vi "AuMT8852B CW Measurement Configuration.vi"(5 "Frequency (2441)":dbl=2441.0, 7 "Set/Get (Set)":enum16{"Set", "Get"}(ring), 8 "error in (no error)":errorcluster, 9 "Frequency units (MHz)":enum16{"Channel", "MHz"}(ring)=enum."MHz", 10 "Gate width (1 ms)":dbl=1.0 format="%.2f", 11 "VISA session":refnum<visa-resource-name>) -> (0 "error out":errorcluster, 1 "Frequency units out":enum16{"Channel", "MHz"}(ring)=enum."MHz", 2 "error code":i32, 3 "VISA session out":refnum<visa-resource-name>, 4 "Frequency out":dbl=2441.0, 6 "Gate width out":dbl=1.0 format="%.2f")   [LabVIEW 2017]
doc: "Anritsu MT8852B Bluetooth Tester\n\nSets the frequency and measurement period for the CW measurement.\n\nINPUTS\nSet/Get - whether the configuration is being sent to or retrieved from the instrument.\nFrequency - frequency at which the CW measurement will be made.\nFrequency units - whether frequency will be read/written as a channel or as a frequency in MHz.\nGate width - measurement period in ms.\n\nOUTPUTS\nFrequency out - current CW measurement frequency.\nFrequency units out - whether frequency is returned as a channel or as a frequency in MHz.\nGate width - current CW measurement period in ms."
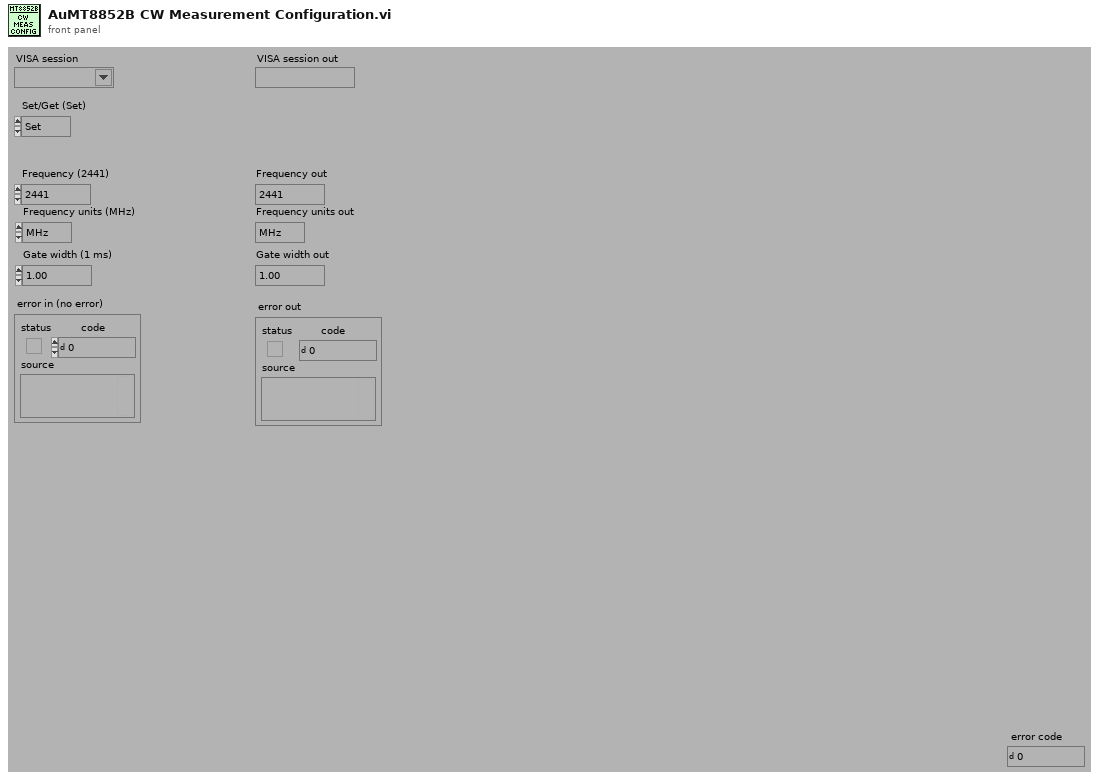
[diagram p1: front panel]
types:
  T1 = enum16{"Simulate", "Range check", "Cache", "Query instrument status"}
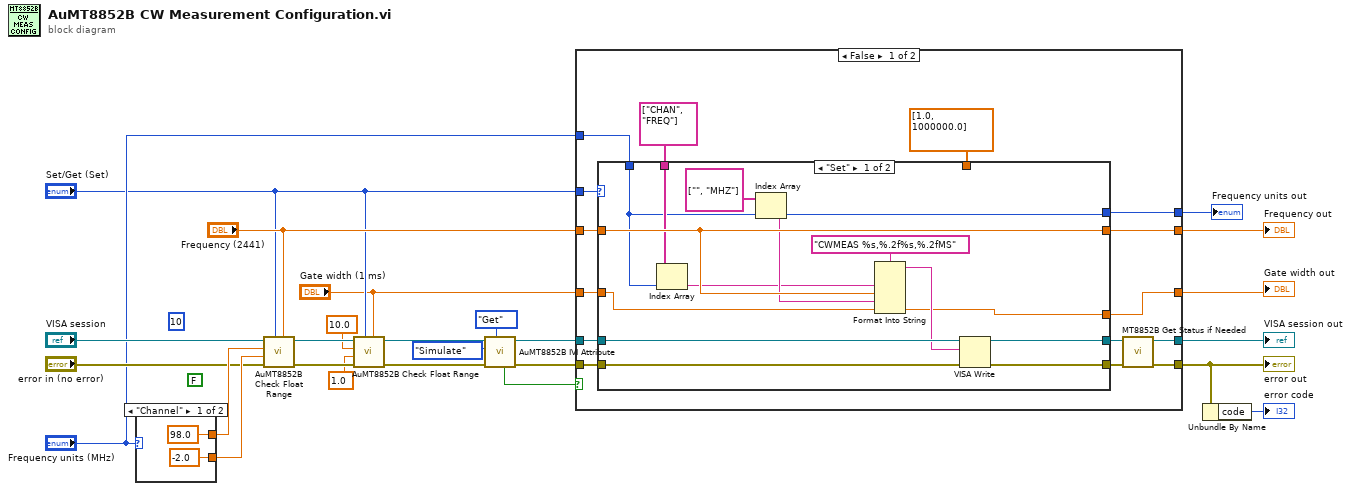
[diagram p0: block diagram]
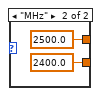
[diagram p2: hidden frame]
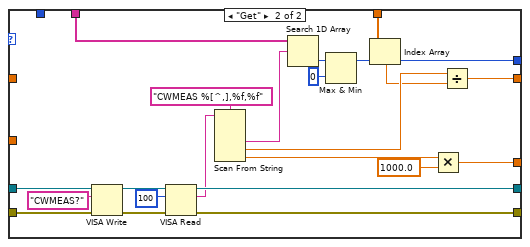
[diagram p3: hidden frame]
diagram:
  (unwired) FALSE ("Check IVI flag first? (T)")
  (unwired) 10 ("Upper limit (1)")
  n1 = case shown="\"Channel\"" "Frequency units (MHz)" {
    tunnel: [98.0 ("Upper limit (1)") 2500.0 ("Upper limit (1)")] -> w15
    tunnel: [-2.0 ("Lower limit (-1)") 2400.0 ("Lower limit (-1)")] -> w14
    frame "Channel" {
    }
    frame "MHz" {
    }
  }
  n2 = call <instrlib>:"AuMT8852B Check Float Range.vi"("Value (0)"="Frequency (2441)", "Set/Get (Set)"="Set/Get (Set)", "error in (no error)"="error in (no error)", "Lower limit (-1)"=w14, "Upper limit (1)"=w15, "VISA session"="VISA session") -> ("error out"=w9:errorcluster, "VISA session out"=w8:refnum<visa-resource-name>)  [unwired: 4 in]
  n3 = call <instrlib>:"AuMT8852B Check Float Range.vi"("Value (0)"="Gate width (1 ms)", "Set/Get (Set)"="Set/Get (Set)", "error in (no error)"=w9, "Lower limit (-1)"=1.0, "Upper limit (1)"=10.0, "VISA session"=w8) -> ("error out"=w6:errorcluster, "VISA session out"=w7:refnum<visa-resource-name>)  [unwired: 4 in]
  n4 = call <instrlib>:"AuMT8852B IVI Attribute.vi"("Set/Get (Set)"=enum16{"Set", "Get"}."Get", "error in (no error)"=w6, "Flag (Simulate)"=T1."Simulate", "VISA session"=w7) -> ("error out"=w23:errorcluster, "VISA session out"=w24:refnum<visa-resource-name>, "Value out"=w20:bool)  [unwired: 5 in]
  n5 = case shown="False" w20 {
    tunnel: "Set/Get (Set)" -> [w44 _]
    tunnel: [w38 w83] -> w18
    tunnel: [w39 w84] -> w25
    tunnel: w24 -> [w43 w84]
    tunnel: w23 -> [w42 w83]
    tunnel: "Frequency (2441)" -> [w37 w82]
    tunnel: [w36 w82] -> w17
    tunnel: "Frequency units (MHz)" -> [w31 w80]
    tunnel: "Gate width (1 ms)" -> [w35 w81]
    tunnel: [w34 w81] -> w10
    tunnel: [w30 w80] -> w1
    frame False {
      n6 = case shown="\"Set\"" w44 {
        tunnel: [w54 w73] -> w40
        tunnel: [w55 w74] -> w41
        tunnel: w43 -> [w57 w79]
        tunnel: w42 -> [w56 w78]
        tunnel: w37 -> [w51 _]
        tunnel: [w51 w72] -> w36
        tunnel: string[] ["CHAN", "FREQ"] ("Array Constant") -> [w47 w64]
        tunnel: w35 -> [w50 _]
        tunnel: [w50 w67] -> w34
        tunnel: w31 -> [w46 _]
        tunnel: dbl[] [1.0, 1000000.0] ("Input Array") -> [_ w59]
        tunnel: [w46 w62] -> w30
        frame "Set" {
          n7 = Index Array(array=w47, index=w46) -> (element=w45:string)
          n8 = Index Array(array=string[] ["", "MHZ"] ("Array Constant"), index=w46) -> (element=w48:string)
          n9 = Format Into String(format string="CWMEAS %s,%.2f%s,%.2fMS" ("Format String"), w45, w51, w48, w50) -> (resulting string=w52:string)  [unwired: 2 in, 1 out]
          n10 = VISA Write(VISA resource name=w57, write buffer=w52, error in (no error)=w56) -> (VISA resource name out=w55:refnum<visa-resource-name>, error out=w54:errorcluster)  [unwired: 1 out]
        }
        frame "Get" {
          n11 = VISA Write(VISA resource name=w79, write buffer="CWMEAS?" ("Format String"), error in (no error)=w78) -> (VISA resource name out=w77:refnum<visa-resource-name>, error out=w75:errorcluster)  [unwired: 1 out]
          n12 = VISA Read(VISA resource name=w77, byte count=u32 100 ("byte count (0)"), error in (no error)=w75) -> (VISA resource name out=w74:refnum<visa-resource-name>, read buffer=w71:string, error out=w73:errorcluster)  [unwired: 1 out]
          n13 = Scan From String(format string="CWMEAS %[^,],%f,%f" ("Format String"), input string=w71) -> (output 1=w63:string, output 2=w69:dbl, output 3=w68:dbl)  [unwired: 5 in, 3 out]
          n14 = Search 1D Array(1D array=w64, element=w63) -> (index of element=w60:i32)  [unwired: 1 in]
          n15 = Max & Min(x=w60, y=0 ("x")) -> (max(x,y)=w62:i32)  [unwired: 1 out]
          n16 = Index Array(array=w59, index=w62) -> (element=w58:dbl)
          n17 = Multiply(x=w68, y=1000.0) -> (x*y=w67:dbl)
          n18 = Divide(x=w69, y=w58) -> (x/y=w72:dbl)
        }
      }
      n19 = call <instrlib>:"MT8852B Get Status if Needed.vi"("error in (no error)"=w40, "VISA session"=w41) -> ("error out"=w38:errorcluster, "VISA session out"=w39:refnum<visa-resource-name>)  [unwired: 8 in]
    }
    frame True {
    }
  }
  "error out" <- w18
  "VISA session out" <- w25
  "Frequency out" <- w17
  "Gate width out" <- w10
  "Frequency units out" <- w1
  n20 = Unbundle By Name(w18) -> ("code"=→"error code":i32)
